vi "LIEB_finalMatos.vi"() -> ()   [LabVIEW 2019]
uses:
  <vilib>/Utility/file.llb/Read Delimited Spreadsheet (DBL).vi
panel:
  in  "JAVA":bool
  in  "SIDES":bool
  out "CHANGES":dbl
  out "Array 3":dbl[](array[numeric])
  out "Array 2":dbl[](array[numeric])
  out "Array":dbl[](array[numeric])
  out "rest":dbl[](array[numeric])
  out "peak -":dbl[](array[numeric])
  out "peak +":dbl[](array[numeric])
  out "Release":bool
  out "Release eye controller  when LED turns RED":bool
  out "Horizontal EOG":dbl[](graph)
  out "Vertical EOG":dbl[](graph)
  in  "STOP":bool
  out "LED":bool
  in  "DOWN":bool
  in  "UP":bool
  in  "L":bool
  in  "R":bool
  # "OCULAR MOVEMENT"
  # "Release eye controller  when LED turns RED"
  # "HORIZONTAL"
  # "VERTICAL"
  # "FRONTAL"
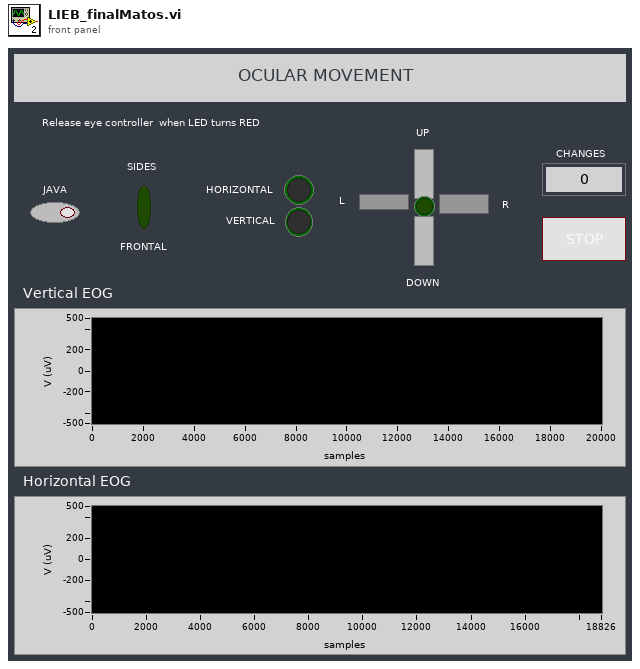
[diagram p1: front panel]
types:
  T1 = enum16{"open", "replace", "create", "open or create", "replace or create", "replace or create with confirmation"}
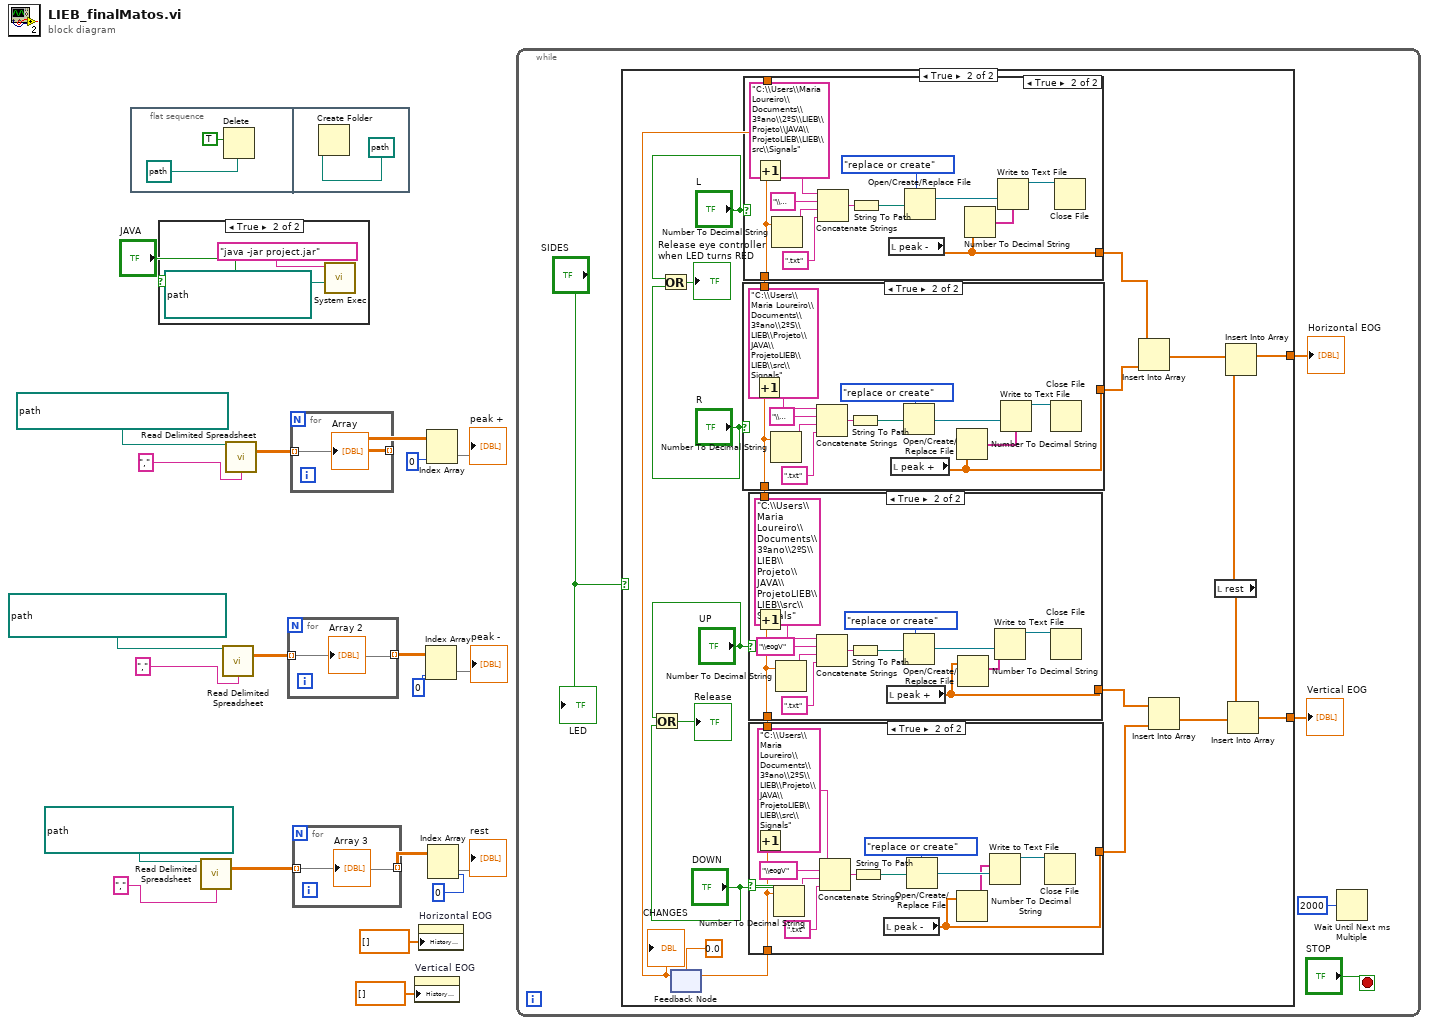
[diagram p0: block diagram]
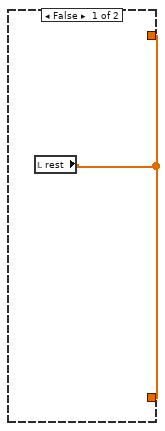
[diagram p3: hidden frame]
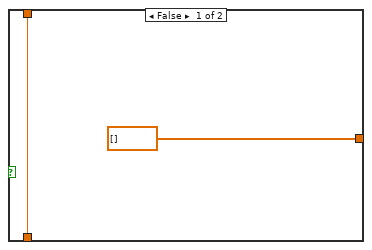
[diagram p4: hidden frame]
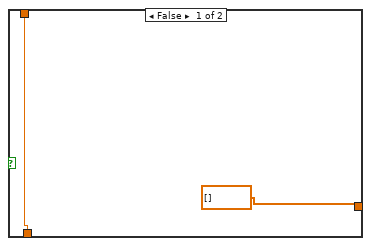
[diagram p5: hidden frame]
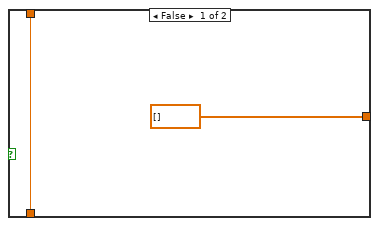
[diagram p6: hidden frame]
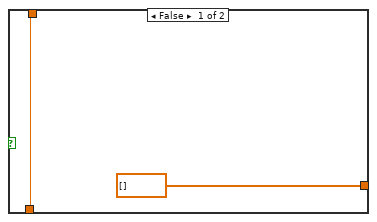
[diagram p7: hidden frame]
diagram:
  n1 = flat-sequence {
    frame #0 {
      n2 = Delete(path (use dialog)=path "C:/Users/Maria Loureiro/Documents/3ºano/2ºS/LIEB/Projeto/JAVA/ProjetoLIEB/LIEB/src/Signals", entire hierarchy (F)=TRUE) -> ()  [unwired: 3 in, 3 out]
    }
    frame #1 {
      n3 = Create Folder(path (use dialog)=path "C:/Users/Maria Loureiro/Documents/3ºano/2ºS/LIEB/Projeto/JAVA/ProjetoLIEB/LIEB/src/Signals") -> ()  [unwired: 2 in, 3 out]
    }
  }
  n4 = case shown="True" "JAVA" {
    frame False {
    }
    frame True {
      n5 = call <vilib>:"System Exec.vi"("working directory"=path "C:/Users/Maria Loureiro/Documents/3ºano/2ºS/LIEB/Projeto/JAVA/ProjetoLIEB/LIEB", "command line"="java -jar project.jar") -> ()  [unwired: 6 in, 4 out]
    }
  }
  n6 = call-poly <vilib>:"Read Delimited Spreadsheet.vi"("file path (dialog if empty)"=path "C:/Users/Maria Loureiro/Documents/3ºano/2ºS/LIEB/Projeto/JAVA/ProjetoLIEB/LIEB/src/repouso.csv" ("Path"), "delimiter (\\t)"="," ("delimiter (\\t)")) -> ("all rows"=w4:dbl[][])  [unwired: 8 in, 5 out]
  n7 = call-poly <vilib>:"Read Delimited Spreadsheet.vi"("file path (dialog if empty)"=path "C:/Users/Maria Loureiro/Documents/3ºano/2ºS/LIEB/Projeto/JAVA/ProjetoLIEB/LIEB/src/piconegativo.csv" ("Path"), "delimiter (\\t)"="," ("delimiter (\\t)")) -> ("all rows"=w8:dbl[][])  [unwired: 8 in, 5 out]
  n8 = call-poly <vilib>:"Read Delimited Spreadsheet.vi"("file path (dialog if empty)"=path "C:/Users/Maria Loureiro/Documents/3ºano/2ºS/LIEB/Projeto/JAVA/ProjetoLIEB/LIEB/src/picopositivo.csv" ("Path"), "delimiter (\\t)"="," ("delimiter (\\t)")) -> ("all rows"=w12:dbl[][])  [unwired: 8 in, 5 out]
  n9 = for {
    tunnel: w8 -> [w27] mode=indexing
    tunnel: [w27] -> w6 mode=indexing
    "Array 2" <- w27
  }
  n10 = for {
    tunnel: w12 -> [w28] mode=indexing
    tunnel: [w28] -> w10 mode=indexing
    "Array" <- w28
  }
  n11 = for {
    tunnel: w4 -> [w29] mode=indexing
    tunnel: [w29] -> w3 mode=indexing
    "Array 3" <- w29
  }
  n12 = property on="Vertical EOG" class="WFChart (strict)"("History Data"=dbl[] []) -> ()  [unwired: 2 in, 2 out]
  n13 = property on="Horizontal EOG" class="WFChart (strict)"("History Data"=dbl[] []) -> ()  [unwired: 2 in, 2 out]
  n14 = Index Array(array=w6, index (col)=0 ("disabled index (col)")) -> (element=→"peak -":dbl[])  [unwired: 1 in]
  n15 = Index Array(array=w10, index (col)=0 ("disabled index (col)")) -> (element=→"peak +":dbl[])  [unwired: 1 in]
  n16 = Index Array(array=w3, index (col)=0 ("disabled index (col)")) -> (element=→"rest":dbl[])  [unwired: 1 in]
  n17 = while {
    stop <- "STOP" stop-if-true
    n18 = case shown="True" "SIDES" {
      tunnel: [w35 w39] -> w33
      tunnel: [w35 w38] -> w31
      frame False {
        n19 = local read "rest"() -> (w35:dbl[])
      }
      frame True {
        n20 = Or(x="UP", y="DOWN") -> (x .or. y?=→"Release":bool)
        n21 = Or(x="L", y="R") -> (x .or. y?=→"Release eye controller  when LED turns RED":bool)
        n22 = feedback #1(0.0) -> (w55:dbl)
        "CHANGES" <- w55
        n23 = case shown="True" "L" {
          tunnel: w55 -> [w103 w116]
          tunnel: [w103 w115] -> w54
          tunnel: [dbl[] [] ("pico -") w104] -> w44
          frame False {
          }
          frame True {
            n24 = Increment(x=w116) -> (x+1=w115:dbl)
            n25 = Number To Decimal String(number=w115) -> (decimal integer string=w112:string)  [unwired: 1 in]
            n26 = Concatenate Strings("C:\\Users\\Maria Loureiro\\Documents\\3ºano\\2ºS\\LIEB\\Projeto\\JAVA\\ProjetoLIEB\\LIEB\\src\\Signals", "\\eogH" ("string"), w112, ".txt" ("string")) -> (w110:string)
            n27 = String To Path(string=w110) -> (path=w109:path)
            n28 = local read "peak -"() -> (w104:dbl[])
            n29 = Open/Create/Replace File(file path (use dialog)=w109, operation (0:open)=T1."replace or create") -> (refnum out=w107:refnum<file>)  [unwired: 4 in, 2 out]
            n30 = Number To Decimal String(number=w104) -> (decimal integer string=w105:string[])  [unwired: 1 in]
            n31 = Write to Text File(file (use dialog)=w107, text=w105) -> (refnum out=w108:refnum<file>)  [unwired: 2 in, 2 out]
            n32 = Close File(refnum=w108) -> ()  [unwired: 1 in, 2 out]
          }
        }
        n33 = case shown="True" "R" {
          tunnel: w54 -> [w88 w101]
          tunnel: [w88 w92] -> w53
          tunnel: [dbl[] [] ("peak +") w90] -> w43
          frame False {
          }
          frame True {
            n34 = Increment(x=w101) -> (x+1=w92:dbl)
            n35 = Number To Decimal String(number=w92) -> (decimal integer string=w99:string)  [unwired: 1 in]
            n36 = Concatenate Strings("C:\\Users\\Maria Loureiro\\Documents\\3ºano\\2ºS\\LIEB\\Projeto\\JAVA\\ProjetoLIEB\\LIEB\\src\\Signals", "\\eogH" ("string"), w99, ".txt" ("string")) -> (w97:string)
            n37 = String To Path(string=w97) -> (path=w96:path)
            n38 = local read "peak +"() -> (w90:dbl[])
            n39 = Open/Create/Replace File(file path (use dialog)=w96, operation (0:open)=T1."replace or create") -> (refnum out=w94:refnum<file>)  [unwired: 4 in, 2 out]
            n40 = Number To Decimal String(number=w90) -> (decimal integer string=w91:string[])  [unwired: 1 in]
            n41 = Write to Text File(file (use dialog)=w94, text=w91) -> (refnum out=w95:refnum<file>)  [unwired: 2 in, 2 out]
            n42 = Close File(refnum=w95) -> ()  [unwired: 1 in, 2 out]
          }
        }
        n43 = case shown="True" "UP" {
          tunnel: w53 -> [w73 w86]
          tunnel: [w73 w77] -> w52
          tunnel: [dbl[] [] ("peak +") w76] -> w42
          frame False {
          }
          frame True {
            n44 = Increment(x=w86) -> (x+1=w77:dbl)
            n45 = Number To Decimal String(number=w77) -> (decimal integer string=w84:string)  [unwired: 1 in]
            n46 = Concatenate Strings("C:\\Users\\Maria Loureiro\\Documents\\3ºano\\2ºS\\LIEB\\Projeto\\JAVA\\ProjetoLIEB\\LIEB\\src\\Signals", "\\eogV" ("string"), w84, ".txt" ("string")) -> (w82:string)
            n47 = String To Path(string=w82) -> (path=w81:path)
            n48 = local read "peak +"() -> (w76:dbl[])
            n49 = Open/Create/Replace File(file path (use dialog)=w81, operation (0:open)=T1."replace or create") -> (refnum out=w79:refnum<file>)  [unwired: 4 in, 2 out]
            n50 = Number To Decimal String(number=w76) -> (decimal integer string=w75:string[])  [unwired: 1 in]
            n51 = Write to Text File(file (use dialog)=w79, text=w75) -> (refnum out=w80:refnum<file>)  [unwired: 2 in, 2 out]
            n52 = Close File(refnum=w80) -> ()  [unwired: 1 in, 2 out]
          }
        }
        n53 = case shown="True" "DOWN" {
          tunnel: [w58 w62] -> w56
          tunnel: w52 -> [w58 w71]
          tunnel: [dbl[] [] ("peak -") w60] -> w41
          frame False {
          }
          frame True {
            n54 = Increment(x=w71) -> (x+1=w62:dbl)
            n55 = Number To Decimal String(number=w62) -> (decimal integer string=w69:string)  [unwired: 1 in]
            n56 = Concatenate Strings("C:\\Users\\Maria Loureiro\\Documents\\3ºano\\2ºS\\LIEB\\Projeto\\JAVA\\ProjetoLIEB\\LIEB\\src\\Signals", "\\eogV" ("string"), w69, ".txt" ("string")) -> (w67:string)
            n57 = String To Path(string=w67) -> (path=w66:path)
            n58 = local read "peak -"() -> (w60:dbl[])
            n59 = Open/Create/Replace File(file path (use dialog)=w66, operation (0:open)=T1."replace or create") -> (refnum out=w64:refnum<file>)  [unwired: 4 in, 2 out]
            n60 = Number To Decimal String(number=w60) -> (decimal integer string=w61:string[])  [unwired: 1 in]
            n61 = Write to Text File(file (use dialog)=w64, text=w61) -> (refnum out=w65:refnum<file>)  [unwired: 2 in, 2 out]
            n62 = Close File(refnum=w65) -> ()  [unwired: 1 in, 2 out]
          }
        }
        n63 = feedback-in #1(w56) -> ()
        n64 = Insert Into Array(array=w44, new element=w43) -> (w40:dbl[])  [unwired: 1 in]
        n65 = Insert Into Array(array=w42, new element=w41) -> (w36:dbl[])  [unwired: 1 in]
        n66 = local read "rest"() -> (w37:dbl[])
        n67 = Insert Into Array(array=w40, new element=w37) -> (w39:dbl[])  [unwired: 1 in]
        n68 = Insert Into Array(array=w37, new element=w36) -> (w38:dbl[])  [unwired: 1 in]
      }
    }
    "Horizontal EOG" <- w33
    "Vertical EOG" <- w31
    n69 = Wait Until Next ms Multiple(millisecond multiple=u32 2000) -> ()  [unwired: 1 out]
    "LED" <- "SIDES"
  }
